vi "Test Auth Service.vi"() -> ()   [LabVIEW 2020]
uses:
  HTTP Server/Trace Log.ctl
  HTTP Server/Trace Item.ctl
  HTTP Server/Processing Step.ctl
  <vilib>/IlluminatedG/IG HTTP Utils/HTTP Utils/Method.ctl
  TestUser/User Init Info.ctl
  TestAuthController/TestAuthController.lvclass
  C:/dev/IlluminatedG/lv-http-server/HTTP Server/Handler/Handler.lvclass
  TestUser/TestUser.lvclass
  C:/dev/IlluminatedG/lv-http-server/HTTP Server/User/User.lvclass
  HTTP Server/InMemoryUserProvider/InMemoryUserProvider.lvclass
  C:/dev/IlluminatedG/lv-http-server/HTTP Server/User Provider/User Provider.lvclass
  HTTP Server/Server/Add Connection Handler.vi
  HTTP Server/Server/Add Request Handler.vi
  HTTP Server/Server/Add Route Handler.vi
  HTTP Server/Server/Add Controller Handler.vi
  HTTP Server/Server/Add Controller.vi
  HTTP Server/Server/Add Response Handler.vi
  HTTP Server/Server/Add Complete Handler.vi
  HTTP Server/Server/Add Exception Handler.vi
  HTTP Server/Connection Handler/Connection Handler.lvclass
  HTTP Server/Request Handler/Request Handler.lvclass
  HTTP Server/Route Handler/Route Handler.lvclass
  HTTP Server/Controller Handler/Controller Handler.lvclass
  HTTP Server/Controller/Controller.lvclass
  HTTP Server/Response Handler/Response Handler.lvclass
  HTTP Server/Complete Handler/Complete Handler.lvclass
  HTTP Server/Exception Handler/Exception Handler.lvclass
  HTTP Server/Server/Server.lvclass
  HTTP Server/Handler/Handler.lvclass
  HTTP Server/RequestTraceLog/RequestTraceLog.lvclass
  HTTP Server/Session/Session.lvclass
  HTTP Server/HTTP Server.lvlib
  <vilib>/IlluminatedG/IG HTTP Utils/HTTP Utils/HTTP Utils.lvlib
panel:
  out "error out":errorcluster
  in  "Debug":bool=TRUE
  in  "Refresh Traces":bool
  out "Traces":T1[](array[typedef]) {"Sending" format="%_6f"; "Expires" format="%<%X %x>T"; "Created" format="%<%X %x>T"; "Waiting" format="%_6f"; "Parsing" format="%_6f"; "Processing" format="%_6f"; "Items"."Time" format="%.6f"; "Items"."Duration" format="%.6f"}
  in  "Port":u16=36987
  # "Request"
  # "Response"
  # "Session"
  # "Auth"
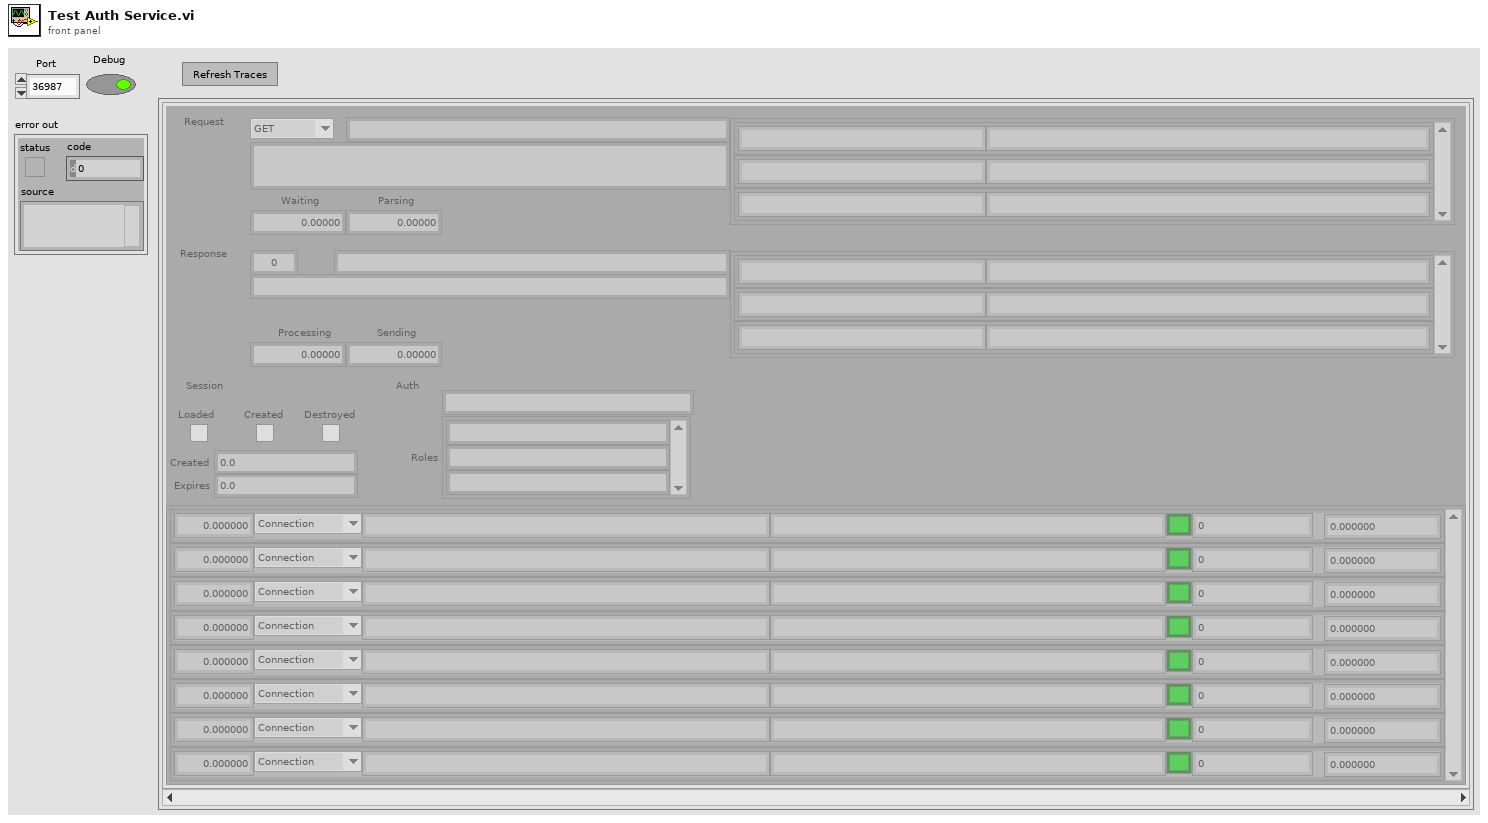
[diagram p1: front panel]
types:
  T1 = typedef "HTTP Server.lvlib/Trace Log.ctl" = cluster{"Items":T2[], "Client":string, "Target":string, "Response Type":string, "Processing":dbl, "Status":u16, "Method":T4, "Content Type":string, "Request Headers":cluster{"Name":string, "Value":string}[], "Parsing":dbl, "Waiting":dbl, "Identity":string, "Loaded":bool, "Created":bool, "Destroyed":bool, "Response Headers":cluster{"Name":string, "Value":string}[], "Created":dbl, "Expires":dbl, "Roles":string[], "Sending":dbl}
  T2 = typedef "HTTP Server.lvlib/Trace Item.ctl" = cluster{"Duration":dbl, "Step":T3, "Class":string, "Info":string, "Status":bool, "Code":i32, "Time":dbl}
  T3 = typedef "HTTP Server.lvlib/Processing Step.ctl" = enum16{"Connection", "Request", "Routing", "Controller Init", "Controller", "Response", "Complete", "Exception"}
  T4 = typedef "HTTP Utils.lvlib/Method.ctl" = enum16{"GET", "HEAD", "POST", "PUT", "DELETE", "CONNECT", "OPTIONS", "TRACE", "PATCH"}
  T5 = typedef "TestUser.lvclass/User Init Info.ctl" = cluster{"Identity":string, "Plain Password":string, "Name":string, "Roles":string[]}
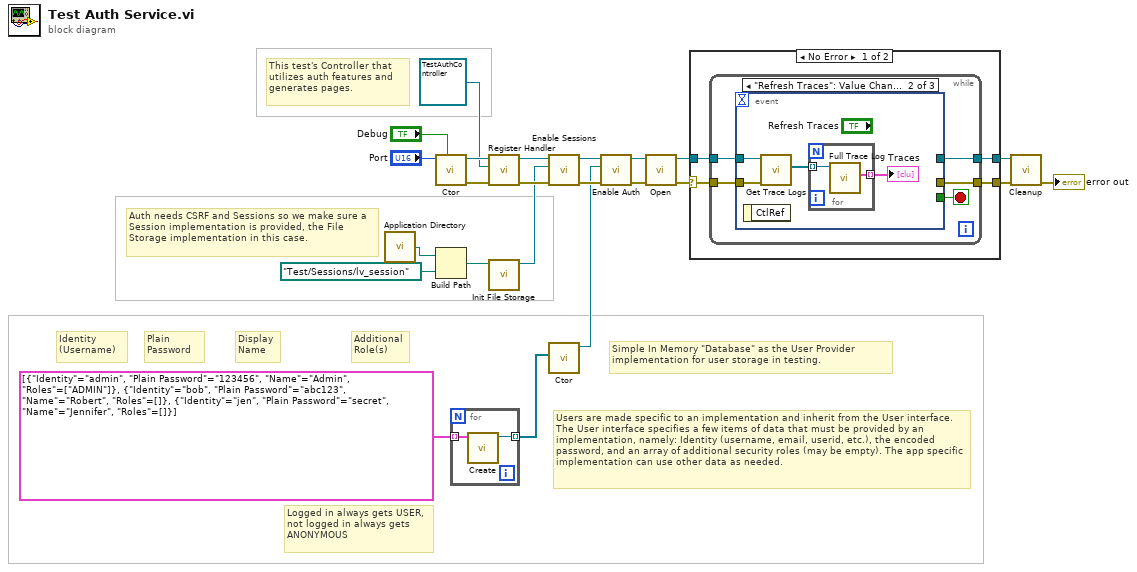
[diagram p0: block diagram]
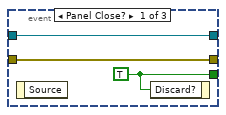
[diagram p2: hidden frame]
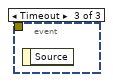
[diagram p3: hidden frame]
diagram:
  # "Users are made specific to an implementation and inherit from the User interface. The User interface specifies a few items of data that must be provided by an implementation, namely: Identity (username, email, userid, etc.), the encoded password, and an array of additional security roles (may be empty). The app specific implementation can use other data as needed."
  # "This test's Controller that utilizes auth features and generates pages."
  # "Logged in always gets USER, not logged in always gets ANONYMOUS"
  # "Additional\nRole(s)"
  # "Display\nName"
  # "Plain\nPassword"
  # "Identity\n(Username)"
  # "Simple In Memory \"Database\" as the User Provider implementation for user storage in testing."
  # "Auth needs CSRF and Sessions so we make sure a Session implementation is provided, the File Storage implementation in this case."
  n1 = call <vilib>:"Application Directory.vi"() -> ("Application Directory"=w12:path)
  n2 = call "Ctor.vi"("Debug (F)"="Debug", "Port (8080)"="Port") -> ("error out"=w14:errorcluster, "Server out"=w15:refnum<class "Server.lvclass">)  [unwired: 8 in]
  n3 = Build Path(base path=w12, name or relative path=path "Test/Sessions/lv_session") -> (appended path=w10:path)
  n4 = for {
    tunnel: T5[] [{"Identity"="admin", "Plain Password"="123456", "Name"="Admin", "Roles"=["ADMIN"]}, {"Identity"="bob", "Plain Password"="abc123", "Name"="Robert", "Roles"=[]}, {"Identity"="jen", "Plain Password"="secret", "Name"="Jennifer", "Roles"=[]}] -> [w25] mode=indexing
    tunnel: [w24] -> w2 mode=indexing
    n5 = call "Create.vi"("User Init Info"=w25) -> ("TestUser out"=w24:refnum<class "TestUser.lvclass">)  [unwired: 9 in, 1 out]
  }
  n6 = call "Register Handler.vi"("error in (no error)"=w14, "Handler"=refnum<class "TestAuthController.lvclass"> refnum ("TestAuthController.lvclass"), "Server in"=w15) -> ("error out"=w8:errorcluster, "Server out"=w9:refnum<class "Server.lvclass">)  [unwired: 7 in]
  n7 = call "Init File Storage.vi"("Session Storage Folder"=w10) -> ("Session out"=w7:refnum<class "Session.lvclass">)  [unwired: 9 in, 1 out]
  n8 = call "Enable Sessions.vi"("error in (no error)"=w8, "Session Implementation"=w7, "Server in"=w9) -> ("error out"=w22:errorcluster, "Server out"=w6:refnum<class "Server.lvclass">)  [unwired: 7 in]
  n9 = call "Ctor.vi"("Starting Users (None)"=w2) -> ("InMemoryUserProvider out"=w1:refnum<class "InMemoryUserProvider.lvclass">)  [unwired: 9 in, 1 out]
  n10 = call "Enable Auth.vi"("error in (no error)"=w22, "User Provider"=w1, "Server in"=w6) -> ("error out"=w4:errorcluster, "Server out"=w5:refnum<class "Server.lvclass">)  [unwired: 7 in]
  n11 = call "Open.vi"("error in (no error)"=w4, "Server in"=w5) -> ("error out"=w18:errorcluster, "Server out"=w19:refnum<class "Server.lvclass">)  [unwired: 8 in]
  n12 = case shown="No Error" w18 {
    selector: w18 -> [w28 w45]
    tunnel: w19 -> [w29 w44]
    tunnel: [w27 w44] -> w17
    tunnel: [w26 w45] -> w16
    frame No Error {
      n13 = while {
        tunnel: w29 -> [w32]
        tunnel: w28 -> [w33]
        tunnel: [w31] -> w27
        tunnel: [w30] -> w26
        stop <- w34 stop-if-true
        n14 = event shown="[1] \"Refresh Traces\": Value Change" {
          selector: _ -> [_ _ _]
          dyn-events: _ -> [_ _ _]
          timeout: _ -> [_ _ _]
          tunnel: [w35 _ _] -> w34
          tunnel: w33 -> [w36 w40 _]
          tunnel: w32 -> [w37 w41 _]
          tunnel: [w37 _ _] -> w31
          tunnel: [w36 _ _] -> w30
          event Panel Close? {
            w35 = TRUE ("Discard?")
            n15 = event-data() -> ()  [unwired: 1 in, 1 out]
            n16 = event-data("Discard?"=w35) -> ()  [unwired: 1 in, 1 out]
          }
          event "Refresh Traces": Value Change {
            n17 = event-data() -> ()  [unwired: 1 in, 1 out]
            n18 = call "Get Trace Logs.vi"("error in (no error)"=w40, "Server in"=w41) -> ("Trace Logs"=w39:refnum<class "RequestTraceLog.lvclass">[])  [unwired: 7 in, 2 out]
            n19 = for {
              tunnel: w39 -> [w43] mode=indexing
              tunnel: [w42] -> w38 mode=indexing
              n20 = call "Full Trace Log.vi"("RequestTraceLog in"=w43) -> ("Trace Log"=w42:T1)  [unwired: 8 in, 2 out]
            }
            "Traces" <- w38
          }
          event Timeout {
            n21 = event-data() -> ()  [unwired: 1 in, 1 out]
          }
        }
      }
    }
    frame Error {
    }
  }
  n22 = call "Cleanup.vi"("error in (no error)"=w16, "Server in"=w17) -> ("error out"=→"error out":errorcluster)  [unwired: 9 in]
